vi "Destroy ID Pool.vi"(8 "error in (no error)":errorcluster, 11 "ID Pool in":refnum<class "ID Pool.lvclass">) -> (0 "error out":errorcluster, 3 "ID Pool out":refnum<class "ID Pool.lvclass">)   [LabVIEW 2017, in "DSF Core.lvlib" / "ID Pool.lvclass"]
uses:
  ID Pool.lvclass
  C:/Git/DSF/Data Sharing Framework/Source/Core/Engine/Classes/Thread Pool/Pool.lvclass
  Pool.lvclass
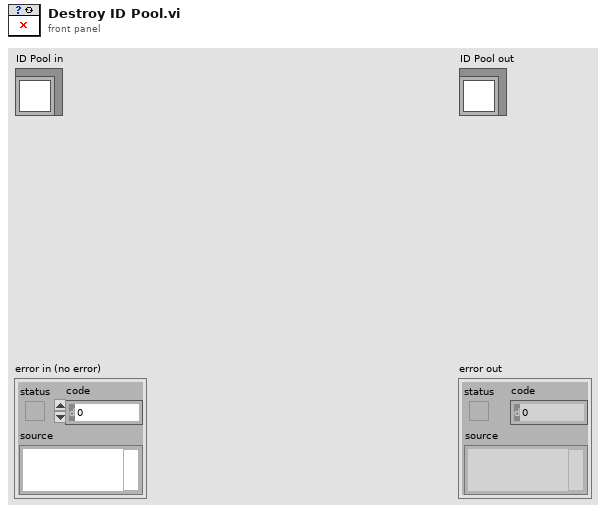
[diagram p1: front panel]
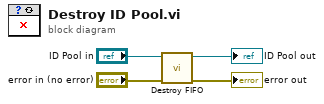
[diagram p0: block diagram]
diagram:
  n1 = call "Destroy FIFO.vi"("error in (no error)"="error in (no error)", "Pool in"="ID Pool in") -> ("error out"=→"error out":errorcluster, "Pool out"=→"ID Pool out":refnum<class "ID Pool.lvclass">)  [unwired: 8 in]
